vi "Get Default Plugin Directories.vi"() -> (3 "Default Plugin Directories":path[](array[path]))   [LabVIEW 2020, in "Plugin Manager.lvlib"]
uses:
  Plugin Manager.lvlib
  <vilib>/Utility/sysdir.llb/System Directory Type.ctl
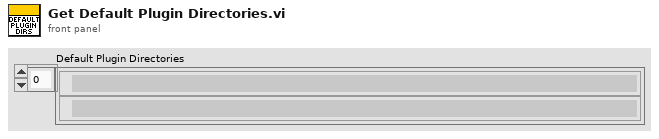
[diagram p1: front panel]
types:
  T1 = typedef "System Directory Type.ctl" = i32
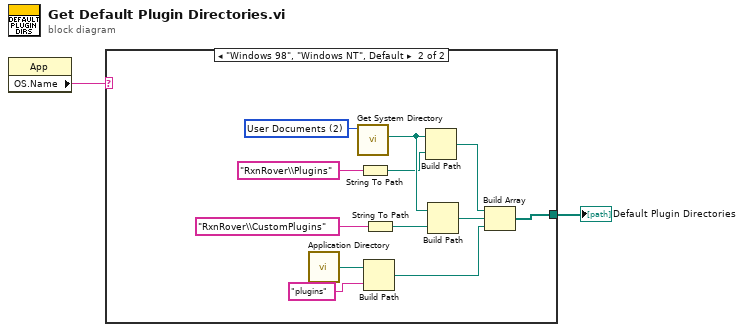
[diagram p0: block diagram]
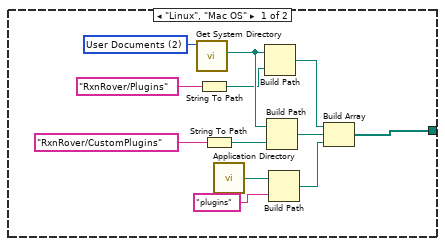
[diagram p2: hidden frame]
diagram:
  n1 = property class="App"() -> ("OS.Name"=w1:string)  [unwired: 2 in, 2 out]
  n2 = case shown="\"Windows 98\", \"Windows NT\", Default" w1 {
    tunnel: [w6 w20] -> w2
    frame "Linux", "Mac OS" {
      w14 = T1 2 items=["User Home"=0, "User Desktop"=1, "User Documents"=2, "User Application Data"=3, "User Preferences"=4, "User Temporary"=5, "Public Documents"=6, "Public Application Data"=7, "Public Preferences"=8, "Public Cache"=13, "System Core Libraries"=9, "System Installed Libraries"=10, "Application Files"=11, "Boot Volume Root"=12] ("system directory type")
      n3 = call <vilib>:"Get System Directory.vi"("system directory type"=w14) -> ("system directory"=w12:path)  [unwired: 10 in]
      n4 = String To Path(string="RxnRover/Plugins" ("name or relative path")) -> (path=w8:path)
      n5 = String To Path(string="RxnRover/CustomPlugins" ("name or relative path")) -> (path=w7:path)
      n6 = call <vilib>:"Application Directory.vi"() -> ("Application Directory"=w5:path)
      n7 = Build Path(base path=w12, name or relative path=w8) -> (appended path=w11:path)
      n8 = Build Path(base path=w12, name or relative path=w7) -> (appended path=w10:path)
      n9 = Build Path(base path=w5, name or relative path="plugins") -> (appended path=w3:path)
      n10 = Build Array(w11, w10, w3) -> (w6:path[])
    }
    frame "Windows 98", "Windows NT", Default {
      w26 = T1 2 items=["User Home"=0, "User Desktop"=1, "User Documents"=2, "User Application Data"=3, "User Preferences"=4, "User Temporary"=5, "Public Documents"=6, "Public Application Data"=7, "Public Preferences"=8, "Public Cache"=13, "System Core Libraries"=9, "System Installed Libraries"=10, "Application Files"=11, "Boot Volume Root"=12] ("system directory type")
      n11 = call <vilib>:"Application Directory.vi"() -> ("Application Directory"=w17:path)
      n12 = call <vilib>:"Get System Directory.vi"("system directory type"=w26) -> ("system directory"=w24:path)  [unwired: 10 in]
      n13 = String To Path(string="RxnRover\\Plugins" ("name or relative path")) -> (path=w19:path)
      n14 = Build Path(base path=w17, name or relative path="plugins") -> (appended path=w15:path)
      n15 = String To Path(string="RxnRover\\CustomPlugins" ("name or relative path")) -> (path=w18:path)
      n16 = Build Path(base path=w24, name or relative path=w19) -> (appended path=w23:path)
      n17 = Build Path(base path=w24, name or relative path=w18) -> (appended path=w22:path)
      n18 = Build Array(w23, w22, w15) -> (w20:path[])
    }
  }
  "Default Plugin Directories" <- w2
